vi "niRFUtil TRC Trace to Waveform (real wfm).vi"(7 "Measurement Trace":T1 format="%.2f") -> (8 "Real Waveform":T2 {"y" min=0 max=127 format="%.2f"; "dx" format="%^.2e"; "x0" format="%^.2e"})   [LabVIEW 2015, in "niRFUtil.lvlib"]
doc: "(c) Copyright 2006, National Instruments, Inc. This VI may not be duplicated, sold, or distributed without written consent from National Instruments."
uses:
  niRFUtil.lvlib
  Includes/niRFUtil INC Real Waveform.ctl
  Includes/niRFUtil INC Real Array.ctl
  Includes/niRFUtil INC Trace.ctl
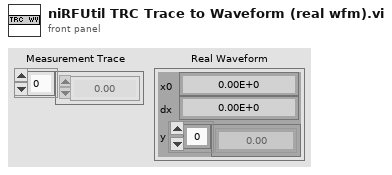
[diagram p1: front panel]
types:
  T1 = typedef "niRFUtil.lvlib/niRFUtil INC Trace.ctl" = sgl[]
  T2 = typedef "niRFUtil.lvlib/niRFUtil INC Real Waveform.ctl" = cluster{"x0":dbl, "dx":dbl, "y":T3}
  T3 = typedef "niRFUtil.lvlib/niRFUtil INC Real Array.ctl" = sgl[]
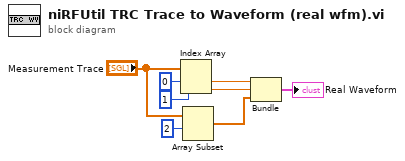
[diagram p0: block diagram]
diagram:
  n1 = Index Array(array="Measurement Trace", index #1=0 ("index"), index #2=1 ("index")) -> (element #1=w6:sgl, element #2=w5:sgl)
  n2 = Array Subset(array="Measurement Trace", index=2) -> (w1:T1)  [unwired: 1 in]
  n3 = Bundle("Numeric"=w6, "Numeric"=w5, w1) -> (→"Real Waveform":cluster{"Numeric":sgl, "Numeric":sgl, T1})  [unwired: 1 out]
